vi "Get Row in Worksheet.vi"(8 "error in":errorcluster, 10 "RowIndex":i32, 11 "Worksheet in":refnum<k24>) -> (0 "error out":errorcluster, 2 "Row out":refnum<k24>, 3 "Worksheet out":refnum<k24>)   [LabVIEW 2019, in "Open Xml.lvlib"]
uses:
  Open Xml.lvlib
  D:/git/Open-Xml-LabVIEW/Source/DocumentFormat.OpenXml.dll
  DocumentFormat.OpenXml.dll
  D:/git/Open-Xml-LabVIEW/Source/DocumentFormat.OpenXml.Framework.dll
  DocumentFormat.OpenXml.Framework.dll
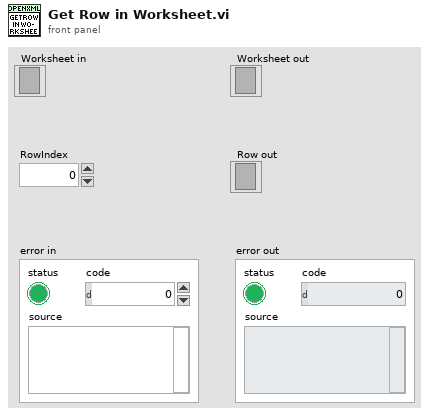
[diagram p1: front panel]
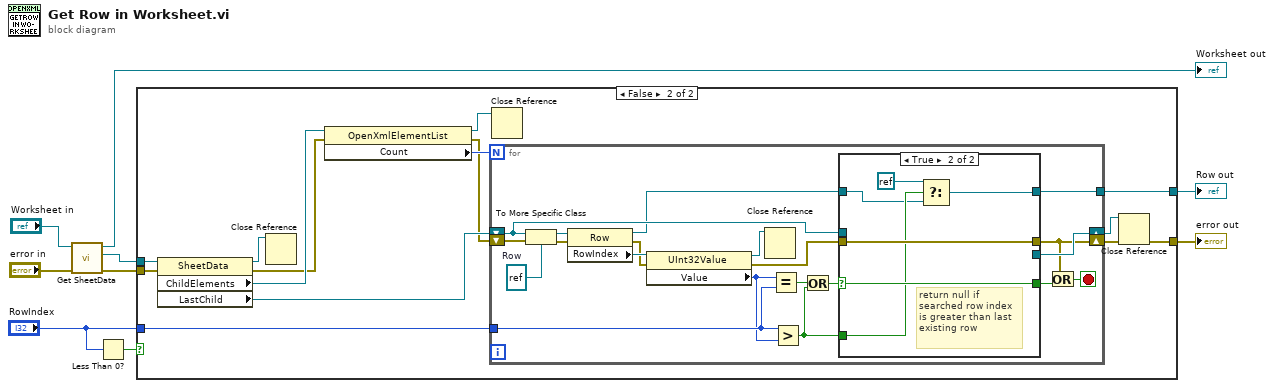
[diagram p0: block diagram]
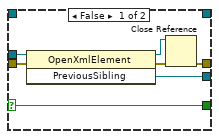
[diagram p3: hidden frame]
diagram:
  n1 = call "Get SheetData.vi"("error in"="error in", "Worksheet in"="Worksheet in") -> ("error out"=w3:errorcluster, "SheetData"=w2:refnum<k24>, "Worksheet out"=→"Worksheet out":refnum<k24>)  [unwired: 7 in]
  n2 = Less Than 0?(x="RowIndex") -> (x < 0?=w9:bool)
  n3 = case shown="False" w9 {
    tunnel: w2 -> [_ w24]
    tunnel: w3 -> [w10 w21]
    tunnel: [_ w18] -> w6
    tunnel: [w10 w14] -> w7
    tunnel: "RowIndex" -> [_ w19]
    frame True {
    }
    frame False {
      n4 = property class="SheetData"(reference=w24, error in=w21) -> (reference out=w16:refnum<k24>, error out=w11:errorcluster, "ChildElements"=w23:refnum<k24>, "LastChild"=w20:refnum<k24>)
      n5 = Close Reference(reference=w16) -> ()  [unwired: 1 in, 1 out]
      n6 = property class="OpenXmlElementList"(reference=w23, error in=w11) -> (reference out=w17:refnum<k24>, error out=w12:errorcluster, "Count"=w22:i32)
      n7 = for {
        N: w22 -> [_]
        shift-right: [w38] -> w13
        shift-left: w20 -> [w39]
        tunnel: w19 -> [w28]
        tunnel: [w34] -> w18
        shift-right: [w37] -> w15
        shift-left: w12 -> [w43]
        stop <- w40 stop-if-true
        w44 = refnum<k24> refnum  # Row
        n8 = To More Specific Class(target class=w44, reference=w39, error in=w43) -> (specific class reference=w41:refnum<k24>, error out=w42:errorcluster)
        n9 = property class="Row"(reference=w41, error in=w42) -> (reference out=w35:refnum<k24>, error out=w31:errorcluster, "RowIndex"=w32:refnum<k24>)
        n10 = property class="UInt32Value"(reference=w32, error in=w31) -> (reference out=w30:refnum<k24>, error out=w29:errorcluster, "Value"=w27:u32)
        n11 = Close Reference(reference=w30) -> ()  [unwired: 1 in, 1 out]
        n12 = Equal?(x=w27, y=w28) -> (x = y?=w33:bool)
        n13 = Greater?(x=w28, y=w27) -> (0:w25:bool)
        n14 = Or(x=w33, y=w25) -> (x .or. y?=w26:bool)
        n15 = case shown="True" w26 {
          selector: w26 -> [w47 w56]
          tunnel: w29 -> [w51 w57]
          tunnel: w39 -> [w50 _]
          tunnel: [w48 _] -> w38
          tunnel: [w45 w57] -> w37
          tunnel: [w47 w56] -> w36
          tunnel: w35 -> [_ w53]
          tunnel: [_ w52] -> w34
          tunnel: w25 -> [_ w55]
          frame False {
            n16 = invoke class="OpenXmlElement" method="PreviousSibling"(reference=w50, error in=w51) -> (reference out=w49:refnum<k24>, error out=w46:errorcluster, "PreviousSibling"=w48:refnum<k24>)  [unwired: 1 in]
            n17 = Close Reference(reference=w49, error in (no error)=w46) -> (error out=w45:errorcluster)
          }
          frame True {
            # "return null if\nsearched row index\nis greater than last\nexisting row"
            n18 = Select(t=refnum<k0> refnum, s=w55, f=w53) -> (s? t:f=w52:refnum<k24>)
          }
        }
        n19 = Or(x=w37, y=w36) -> (x .or. y?=w40:bool)
      }
      n20 = Close Reference(reference=w17) -> ()  [unwired: 1 in, 1 out]
      n21 = Close Reference(reference=w13, error in (no error)=w15) -> (error out=w14:errorcluster)
    }
  }
  "error out" <- w7
  "Row out" <- w6
